vi "Lector de temperatura (subvi).vi"(3 "read buffer":string) -> (0 "T1":dbl caption="Temperatura ambiente" format="%#_4g", 1 "T2":dbl caption="Temperatura del liquido" format="%#_4g")   [LabVIEW 2017]
doc: "Este vi recibe el paquete de datos de la temperatura enviados por el Arduino y los separa en temperatura ambiente y temperatura del liquido."
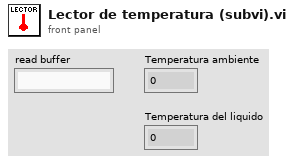
[diagram p1: front panel]
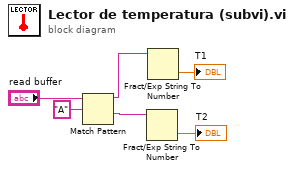
[diagram p0: block diagram]
diagram:
  n1 = Match Pattern(string="read buffer", regular expression="A") -> (before substring=w3:string, after substring=w4:string)  [unwired: 1 in, 2 out]
  n2 = Fract/Exp String To Number(string=w4) -> (number=→"T2":dbl)  [unwired: 3 in, 1 out]
  n3 = Fract/Exp String To Number(string=w3) -> (number=→"T1":dbl)  [unwired: 3 in, 1 out]
